vi "ezAFM Practice 1.3.vi"() -> ()   [LabVIEW 2015]
uses:
  D:/LabVIEW for ezAFM/LV-PGC 2019-05a/Special Equipment/ezAFM/NMI Integration Code/ezCommander.dll
  LabVIEW for ezAFM/LV-PGC 2019-05a/Special Equipment/ezAFM/NMI Integration Code/ezCommander.dll
  LabVIEW for ezAFM/LV-PGC 2019-05a/Universal vi's/Global Variables/Globals-EasyAFM.vi
panel:
  in  "Main Menu":enum32{"Navigation", "Scanning"}(tab)
  out "Status":string
  in  "APPROACH":bool
  in  "RETRACT":bool
  out "Retracting":bool
  out "Approaching":bool
  out "Scanning":bool
  in  "UP":bool
  in  "DOWN":bool
  in  "RIGHT":bool
  in  "LEFT":bool
  in  "Motor Speed":dbl
  in  "Step Size":dbl
  in  "Angle":dbl
  in  "THETA":bool
  out "ezAFM Connected":bool
  out "ezAFM Status":dbl
  out "XY Position":dbl[](array[numeric])
  in  "RESET":bool
  in  "MOVE":bool
  in  "Current Device":string(combo)
  in  "Target Device":string(combo)
  out "XYZ Motor Position":dbl[](array[numeric])
  out "Tip Approached?":bool
  in  "UPDATE DEVICE":bool
  out "Scan Spot":string
  out "Current Device to Scan":string
  in  "Leads":string(combo)
  in  "Device":string(combo)
  in  "Chip":string
  in  "BEGIN SCAN":bool
  in  "Image Resolution":u16(ring)=64 items=["32"=32, "64"=64, "128"=128, "256"=256, "1024"=1024, "2048"=2048]
  out "XY Vector":dbl[](array[numeric])
  in  "QUIT":bool
  # "Use Arrow Keys to manually\nmove the XY Motor"
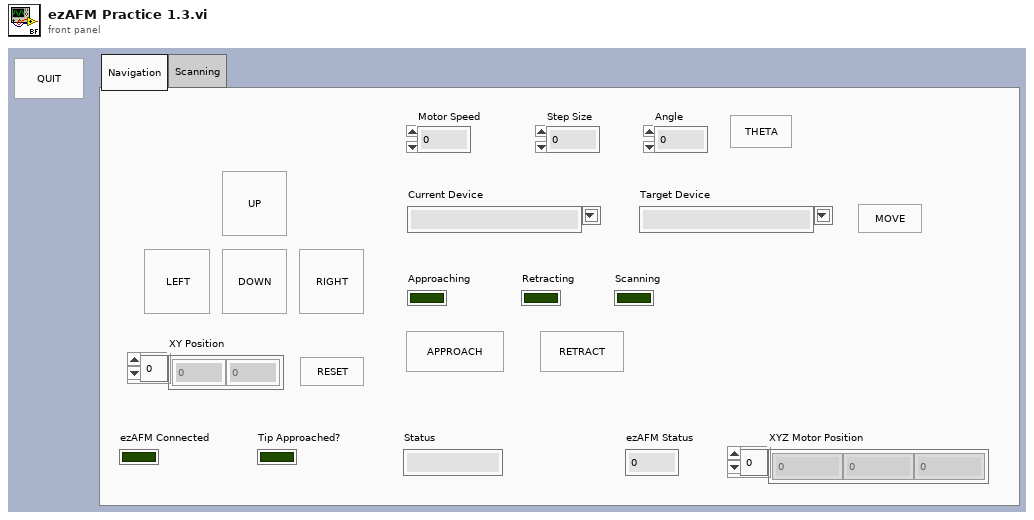
[diagram p1: front panel]
types:
  T1 = typedef "eventvkey.ctl" = enum16{"ASCII", "Enter", "Return", "Shift", "Ctrl", "Alt", "Cmd", "Opt", "Caps", "NumLock", "Clear", "Break", "Up", "Down", "Left", "Right", "Insert", "Delete", "Home", "End", "PageUp", "PageDown", "Escape", "Help", "Pause", "ScrollLock", "F1", "F2", "F3", "F4", "F5", "F6", "F7", "F8", "F9", "F10", "F11", "F12", "F13", "F14", "F15", "F16", "F17", "F18", "F19", "F20", "F21", "F22", "F23", "F24", "Play", "VolumeUp", "VolumeDown", "Mute", "Two Byte Char"}
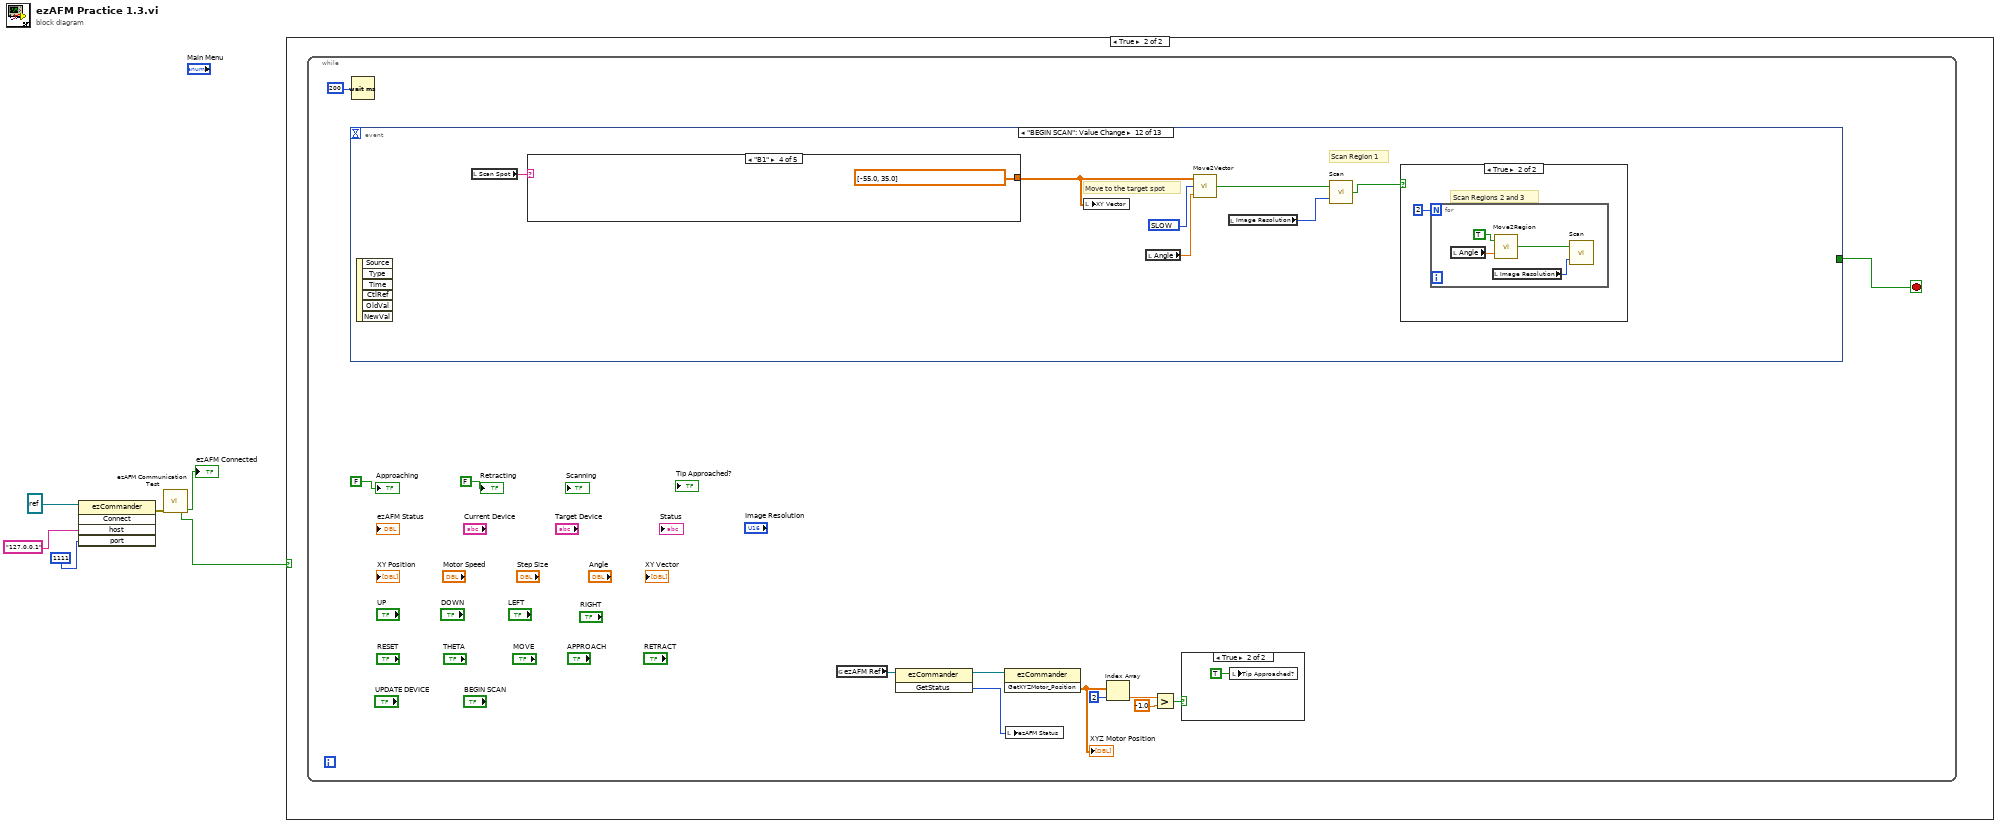
[diagram p0: block diagram]
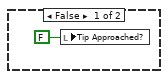
[diagram p3: hidden frame]
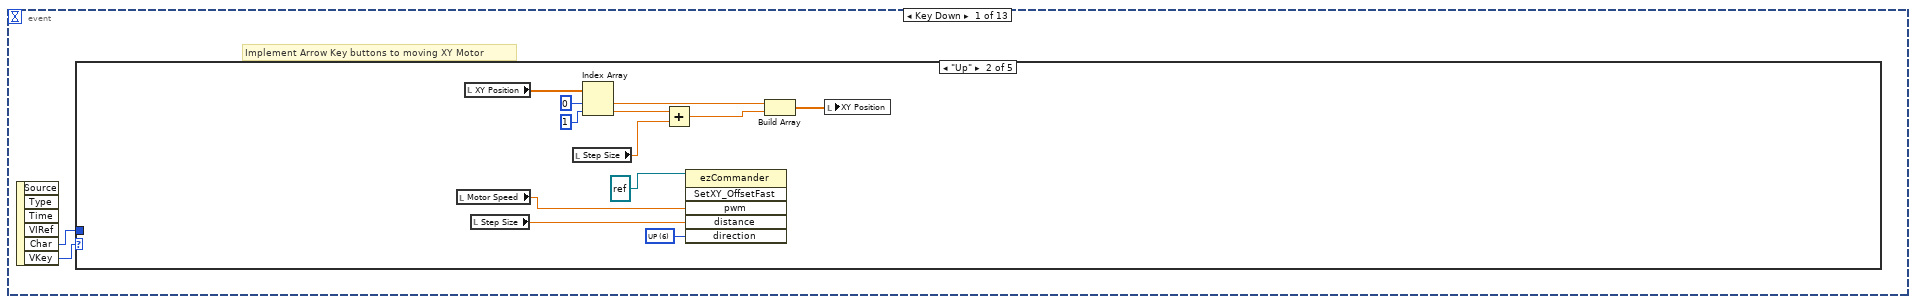
[diagram p4: hidden frame]
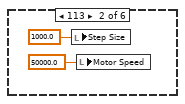
[diagram p6: hidden frame]
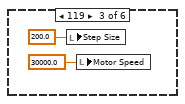
[diagram p7: hidden frame]
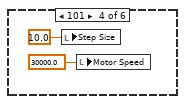
[diagram p8: hidden frame]
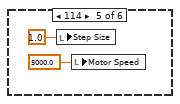
[diagram p9: hidden frame]
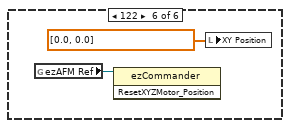
[diagram p10: hidden frame]
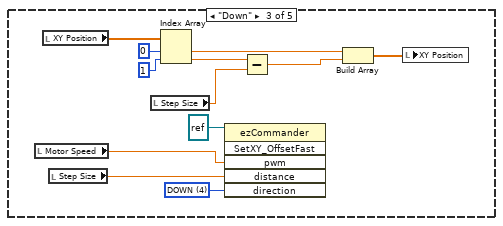
[diagram p11: hidden frame]
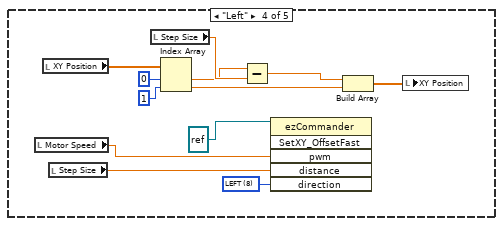
[diagram p12: hidden frame]
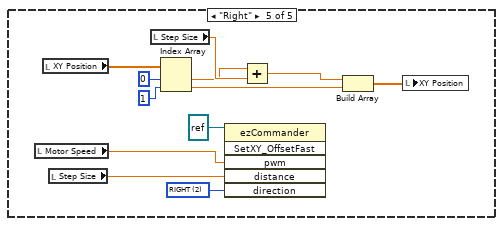
[diagram p13: hidden frame]
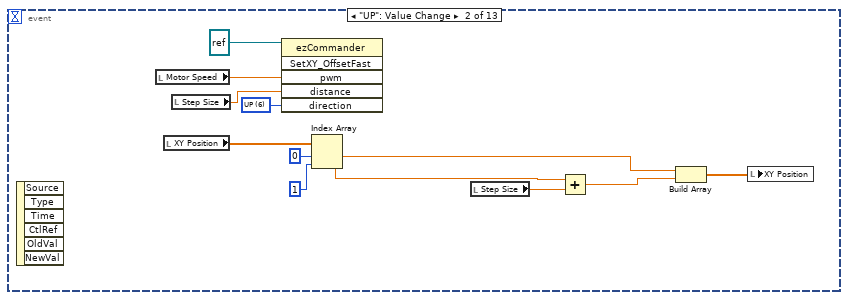
[diagram p14: hidden frame]
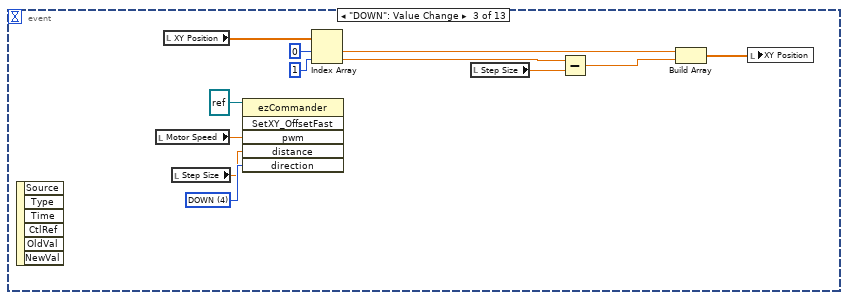
[diagram p15: hidden frame]
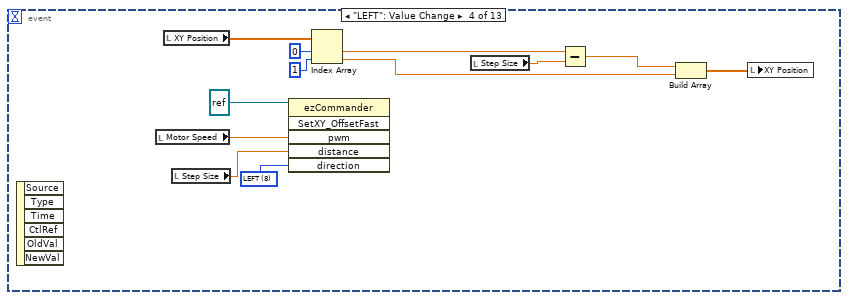
[diagram p16: hidden frame]
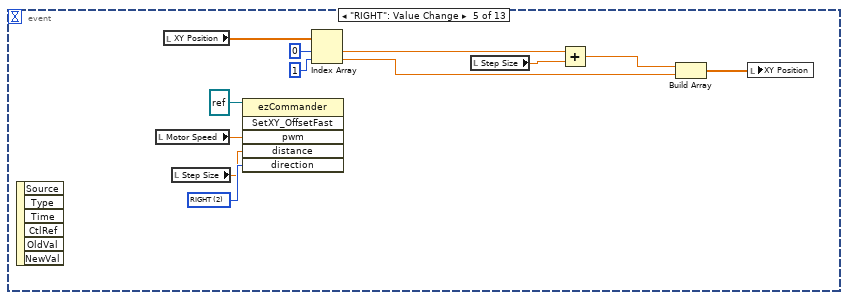
[diagram p17: hidden frame]
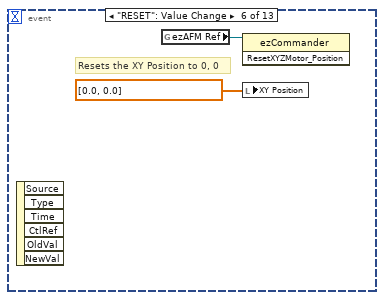
[diagram p18: hidden frame]
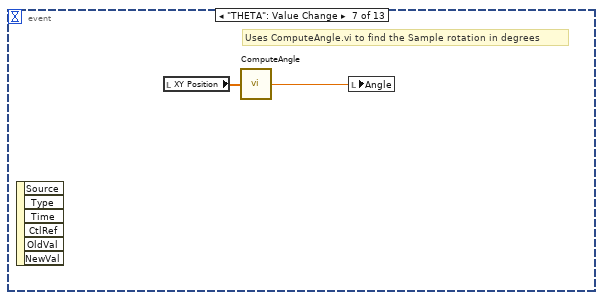
[diagram p19: hidden frame]
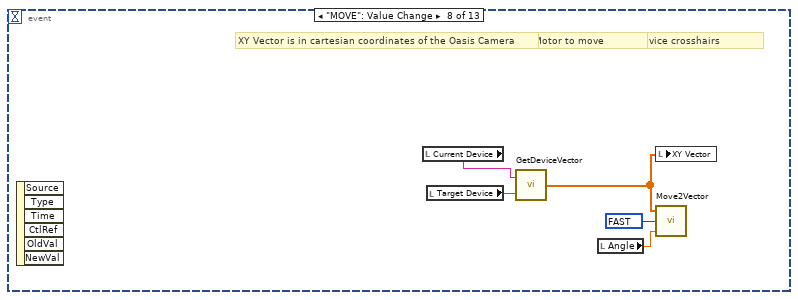
[diagram p20: hidden frame]
diagram:
  n1 = invoke class="ezCommander" method="Connect"(reference=refnum<k24> refnum ("ezAFM Ref"), "host"="127.0.0.1", "port"=1111) -> (error out=w4:errorcluster)  [unwired: 2 in, 4 out]
  n2 = call "ezAFM Communication Test.vi"("error in"=w4) -> ("ezAFM COM status"=w1:bool)  [unwired: 3 in, 3 out]
  "ezAFM Connected" <- w1
  n3 = case shown="True" w1 {
    frame False {
    }
    frame True {
      n4 = while {
        stop <- w17 stop-if-true
        n5 = event shown="[11] \"BEGIN SCAN\": Value Change" {
          selector: _ -> [_ _ _ _ _ _ _ _ _ _ _ _ _]
          dyn-events: _ -> [_ _ _ _ _ _ _ _ _ _ _ _ _]
          timeout: _ -> [_ _ _ _ _ _ _ _ _ _ _ _ _]
          tunnel: [_ _ _ _ _ _ _ _ _ _ _ _ "QUIT"] -> w17
          event Key Down {
            # "Implement Arrow Key buttons to moving XY Motor"
            n6 = event-data() -> ("Char"=w20:i16, "VKey"=w21:T1)  [unwired: 1 in, 4 out]
            n7 = case shown="\"Up\"" w21 {
              tunnel: w20 -> [w22 _ _ _ _]
              frame "ASCII", Default {
                # "Uses 'z' to reset XY Position and XYZ Motor Position"
                # "Uses 'q', 'w', 'e', 'r' keys to set different modes of movement\nAdjusts Motor Speed and Step Size"
                n8 = case shown="0, Default" w22 {
                  frame 0, Default {
                  }
                  frame 113 {
                    n9 = local write "Step Size"(1000.0 ("Step Size")) -> ()
                    n10 = local write "Motor Speed"(50000.0 ("Motor Speed")) -> ()
                  }
                  frame 119 {
                    n11 = local write "Step Size"(200.0 ("Step Size")) -> ()
                    n12 = local write "Motor Speed"(30000.0 ("Motor Speed")) -> ()
                  }
                  frame 101 {
                    n13 = local write "Step Size"(10.0 ("Step Size")) -> ()
                    n14 = local write "Motor Speed"(30000.0 ("Motor Speed")) -> ()
                  }
                  frame 114 {
                    n15 = local write "Step Size"(1.0 ("Step Size")) -> ()
                    n16 = local write "Motor Speed"(5000.0 ("Motor Speed")) -> ()
                  }
                  frame 122 {
                    n17 = global read "Globals-EasyAFM.vi" "ezAFM Ref"() -> (w31:refnum<k24>)
                    n18 = invoke class="ezCommander" method="ResetXYZMotor_Position"(reference=w31) -> ()  [unwired: 2 in, 3 out]
                    n19 = local write "XY Position"(dbl[] [0.0, 0.0] ("XY Position")) -> ()
                  }
                }
              }
              frame "Up" {
                w43 = u16 6 items=["UP"=6, "DOWN"=4, "LEFT"=8, "RIGHT"=2]
                n20 = local read "Motor Speed"() -> (w42:dbl)
                n21 = local read "XY Position"() -> (w40:dbl[])
                n22 = local read "Step Size"() -> (w41:dbl)
                n23 = local read "Step Size"() -> (w37:dbl)
                n24 = Index Array(array=w40, index #1=0 ("index"), index #2=1 ("index")) -> (element #1=w35:dbl, element #2=w36:dbl)
                n25 = Add(x=w36, y=w37) -> (x+y=w34:dbl)
                n26 = invoke class="ezCommander" method="SetXY_OffsetFast"(reference=refnum<k24> refnum ("ezAFM Ref"), "pwm"=w42, "distance"=w41, "direction"=w43) -> ()  [unwired: 2 in, 6 out]
                n27 = Build Array(w35, w34) -> (w33:dbl[])
                n28 = local write "XY Position"(w33) -> ()
              }
              frame "Down" {
                w53 = u16 4 items=["UP"=6, "DOWN"=4, "LEFT"=8, "RIGHT"=2]
                n29 = local read "Motor Speed"() -> (w55:dbl)
                n30 = local read "XY Position"() -> (w47:dbl[])
                n31 = local read "Step Size"() -> (w54:dbl)
                n32 = local read "Step Size"() -> (w46:dbl)
                n33 = Index Array(array=w47, index #1=0 ("index"), index #2=1 ("index")) -> (element #1=w49:dbl, element #2=w50:dbl)
                n34 = invoke class="ezCommander" method="SetXY_OffsetFast"(reference=refnum<k24> refnum ("ezAFM Ref"), "pwm"=w55, "distance"=w54, "direction"=w53) -> ()  [unwired: 2 in, 6 out]
                n35 = Subtract(x=w50, y=w46) -> (x-y=w48:dbl)
                n36 = Build Array(w49, w48) -> (w45:dbl[])
                n37 = local write "XY Position"(w45) -> ()
              }
              frame "Left" {
                w67 = u16 8 items=["UP"=6, "DOWN"=4, "LEFT"=8, "RIGHT"=2]
                n38 = local read "Motor Speed"() -> (w65:dbl)
                n39 = local read "XY Position"() -> (w61:dbl[])
                n40 = local read "Step Size"() -> (w66:dbl)
                n41 = local read "Step Size"() -> (w62:dbl)
                n42 = Index Array(array=w61, index #1=0 ("index"), index #2=1 ("index")) -> (element #1=w59:dbl, element #2=w57:dbl)
                n43 = Subtract(x=w59, y=w62) -> (x-y=w58:dbl)
                n44 = invoke class="ezCommander" method="SetXY_OffsetFast"(reference=refnum<k24> refnum ("ezAFM Ref"), "pwm"=w65, "distance"=w66, "direction"=w67) -> ()  [unwired: 2 in, 6 out]
                n45 = Build Array(w58, w57) -> (w60:dbl[])
                n46 = local write "XY Position"(w60) -> ()
              }
              frame "Right" {
                w79 = u16 2 items=["UP"=6, "DOWN"=4, "LEFT"=8, "RIGHT"=2]
                n47 = local read "Motor Speed"() -> (w78:dbl)
                n48 = local read "XY Position"() -> (w73:dbl[])
                n49 = local read "Step Size"() -> (w77:dbl)
                n50 = local read "Step Size"() -> (w72:dbl)
                n51 = Index Array(array=w73, index #1=0 ("index"), index #2=1 ("index")) -> (element #1=w71:dbl, element #2=w69:dbl)
                n52 = invoke class="ezCommander" method="SetXY_OffsetFast"(reference=refnum<k24> refnum ("ezAFM Ref"), "pwm"=w78, "distance"=w77, "direction"=w79) -> ()  [unwired: 2 in, 6 out]
                n53 = Add(x=w71, y=w72) -> (x+y=w70:dbl)
                n54 = Build Array(w70, w69) -> (w74:dbl[])
                n55 = local write "XY Position"(w74) -> ()
              }
            }
          }
          event "UP": Value Change {
            w91 = u16 6 items=["UP"=6, "DOWN"=4, "LEFT"=8, "RIGHT"=2]
            n56 = event-data() -> ()  [unwired: 1 in, 6 out]
            n57 = local read "Motor Speed"() -> (w84:dbl)
            n58 = local read "XY Position"() -> (w85:dbl[])
            n59 = local read "Step Size"() -> (w83:dbl)
            n60 = invoke class="ezCommander" method="SetXY_OffsetFast"(reference=refnum<k24> refnum ("ezAFM Ref"), "pwm"=w84, "distance"=w83, "direction"=w91) -> ()  [unwired: 2 in, 6 out]
            n61 = Index Array(array=w85, index #1=0 ("index"), index #2=1 ("index")) -> (element #1=w87:dbl, element #2=w88:dbl)
            n62 = local read "Step Size"() -> (w82:dbl)
            n63 = Add(x=w88, y=w82) -> (x+y=w86:dbl)
            n64 = Build Array(w87, w86) -> (w81:dbl[])
            n65 = local write "XY Position"(w81) -> ()
          }
          event "DOWN": Value Change {
            w103 = u16 4 items=["UP"=6, "DOWN"=4, "LEFT"=8, "RIGHT"=2]
            n66 = event-data() -> ()  [unwired: 1 in, 6 out]
            n67 = local read "Motor Speed"() -> (w96:dbl)
            n68 = local read "XY Position"() -> (w95:dbl[])
            n69 = local read "Step Size"() -> (w97:dbl)
            n70 = invoke class="ezCommander" method="SetXY_OffsetFast"(reference=refnum<k24> refnum ("ezAFM Ref"), "pwm"=w96, "distance"=w97, "direction"=w103) -> ()  [unwired: 2 in, 6 out]
            n71 = Index Array(array=w95, index #1=0 ("index"), index #2=1 ("index")) -> (element #1=w99:dbl, element #2=w100:dbl)
            n72 = local read "Step Size"() -> (w94:dbl)
            n73 = Subtract(x=w100, y=w94) -> (x-y=w98:dbl)
            n74 = Build Array(w99, w98) -> (w93:dbl[])
            n75 = local write "XY Position"(w93) -> ()
          }
          event "LEFT": Value Change {
            w115 = u16 8 items=["UP"=6, "DOWN"=4, "LEFT"=8, "RIGHT"=2]
            n76 = event-data() -> ()  [unwired: 1 in, 6 out]
            n77 = local read "Motor Speed"() -> (w105:dbl)
            n78 = local read "XY Position"() -> (w108:dbl[])
            n79 = local read "Step Size"() -> (w107:dbl)
            n80 = invoke class="ezCommander" method="SetXY_OffsetFast"(reference=refnum<k24> refnum ("ezAFM Ref"), "pwm"=w105, "distance"=w107, "direction"=w115) -> ()  [unwired: 2 in, 6 out]
            n81 = Index Array(array=w108, index #1=0 ("index"), index #2=1 ("index")) -> (element #1=w112:dbl, element #2=w110:dbl)
            n82 = local read "Step Size"() -> (w106:dbl)
            n83 = Subtract(x=w112, y=w106) -> (x-y=w111:dbl)
            n84 = Build Array(w111, w110) -> (w109:dbl[])
            n85 = local write "XY Position"(w109) -> ()
          }
          event "RIGHT": Value Change {
            w127 = u16 2 items=["UP"=6, "DOWN"=4, "LEFT"=8, "RIGHT"=2]
            n86 = event-data() -> ()  [unwired: 1 in, 6 out]
            n87 = local read "Motor Speed"() -> (w120:dbl)
            n88 = local read "XY Position"() -> (w119:dbl[])
            n89 = local read "Step Size"() -> (w121:dbl)
            n90 = invoke class="ezCommander" method="SetXY_OffsetFast"(reference=refnum<k24> refnum ("ezAFM Ref"), "pwm"=w120, "distance"=w121, "direction"=w127) -> ()  [unwired: 2 in, 6 out]
            n91 = Index Array(array=w119, index #1=0 ("index"), index #2=1 ("index")) -> (element #1=w124:dbl, element #2=w122:dbl)
            n92 = local read "Step Size"() -> (w118:dbl)
            n93 = Add(x=w124, y=w118) -> (x+y=w123:dbl)
            n94 = Build Array(w123, w122) -> (w117:dbl[])
            n95 = local write "XY Position"(w117) -> ()
          }
          event "RESET": Value Change {
            # "Resets the XY Position to 0, 0"
            n96 = event-data() -> ()  [unwired: 1 in, 6 out]
            n97 = global read "Globals-EasyAFM.vi" "ezAFM Ref"() -> (w129:refnum<k24>)
            n98 = invoke class="ezCommander" method="ResetXYZMotor_Position"(reference=w129) -> ()  [unwired: 2 in, 3 out]
            n99 = local write "XY Position"(dbl[] [0.0, 0.0] ("XY Position")) -> ()
          }
          event "THETA": Value Change {
            # "Uses ComputeAngle.vi to find the Sample rotation in degrees"
            n100 = event-data() -> ()  [unwired: 1 in, 6 out]
            n101 = local read "XY Position"() -> (w132:dbl[])
            n102 = call "ComputeAngle.vi"("XY Vector"=w132) -> ("Angle"=w131:dbl)
            n103 = local write "Angle"(w131) -> ()
          }
          event "MOVE": Value Change {
            w133 = u16 50000 items=["SLOW"=5000, "MEDIUM"=30000, "FAST"=50000]
            # "XY Vector is in cartesian coordinates of the Oasis Camera"
            # "Inputs the XY Vector into Move2Vector.vi to command the XY Motor to move"
            # "Uses Move2Device.vi to find the XY Vector between the Current Device and Target Device crosshairs"
            n104 = event-data() -> ()  [unwired: 1 in, 6 out]
            n105 = local read "Current Device"() -> (w136:string)
            n106 = local read "Target Device"() -> (w135:string)
            n107 = call "GetDeviceVector.vi"("Target Device"=w135, "Current Device"=w136) -> ("XY Vector"=w134:dbl[])
            n108 = local read "Angle"() -> (w137:dbl)
            n109 = local write "XY Vector"(w134) -> ()
            n110 = call "Move2Vector.vi"("Angle"=w137, "Motor Speed"=w133, "XY Vector"=w134) -> ()  [unwired: 1 out]
          }
          event "APPROACH": Value Change {
            w138 = TRUE
            n111 = event-data() -> ()  [unwired: 1 in, 6 out]
            n112 = local write "Approaching"(w138) -> ()
            n113 = call "AutoLand&Approach.vi"("Approaching?"=w138) -> ("Finished?"=w139:bool)
            n114 = local write "Tip Approached?"(w139) -> ()
          }
          event "RETRACT": Value Change {
            w140 = TRUE ("Retracting?")
            n115 = event-data() -> ()  [unwired: 1 in, 6 out]
            n116 = local write "Retracting"(w140) -> ()
            n117 = call "Retract.vi"("Number of Cycles"=10, "Retracting?"=w140) -> ("Finished?"=w142:bool)
            n118 = Not(x=w142) -> (.not. x?=w141:bool)
            n119 = local write "Tip Approached?"(w141) -> ()
          }
          event "UPDATE DEVICE": Value Change {
            n120 = event-data() -> ()  [unwired: 1 in, 6 out]
            n121 = local read "Device"() -> (w145:string)
            n122 = local read "Leads"() -> (w144:string)
            n123 = Concatenate Strings("Chip", w145, w144) -> (→"Current Device to Scan":string)
            n124 = case shown="\"abcde\"" "Leads" {
              tunnel: ["None" "A" ("string") "B" ("string")] -> w146
              frame "None", Default {
              }
              frame "abcde" {
              }
              frame "efgh" {
              }
            }
            n125 = String Length(string="Device") -> (length=w149:i32)
            n126 = Decrement(x=w149) -> (x-1=w148:i32)
            n127 = String Subset(string="Device", offset (0)=w148) -> (substring=w147:string)  [unwired: 1 in]
            n128 = case shown="\"1\", \"3\"" w147 {
              tunnel: w146 -> [w155 w157 w160]
              tunnel: [w155 w156 w159] -> w152
              frame "None", Default {
              }
              frame "0", "2" {
                n129 = Concatenate Strings(w157, "1" ("string")) -> (w156:string)
              }
              frame "1", "3" {
                n130 = Concatenate Strings(w160, "2" ("string")) -> (w159:string)
              }
            }
            "Scan Spot" <- w152
          }
          event "BEGIN SCAN": Value Change {
            w169 = u16 5000 items=["SLOW"=5000, "MEDIUM"=30000, "FAST"=50000]
            # "Scan Region 1"
            # "Move to the target spot"
            n131 = event-data() -> ()  [unwired: 1 in, 6 out]
            n132 = local read "Scan Spot"() -> (w170:string)
            n133 = case shown="\"B1\"" w170 {
              tunnel: [dbl[] [0.0, 0.0] dbl[] [-73.0, 35.0] dbl[] [-73.0, -59.0] dbl[] [-55.0, 35.0] dbl[] [-55.0, -59.0]] -> w166
              frame "None", Default {
              }
              frame "A1" {
              }
              frame "A2" {
              }
              frame "B1" {
              }
              frame "B2" {
              }
            }
            n134 = local write "XY Vector"(w166) -> ()
            n135 = local read "Angle"() -> (w168:dbl)
            n136 = call "Move2Vector.vi"("Angle"=w168, "Motor Speed"=w169, "XY Vector"=w166) -> ("Finished?"=w171:bool)
            n137 = local read "Image Resolution"() -> (w165:u16)
            n138 = call "Scan.vi"("Image Resolution"=w165, "Scanning"=w171) -> ("Finished?"=w167:bool)
            n139 = case shown="True" w167 {
              frame False {
              }
              frame True {
                # "Scan Regions 2 and 3"
                n140 = for {
                  N: 2 -> [_]
                  n141 = local read "Angle"() -> (w176:dbl)
                  n142 = local read "Image Resolution"() -> (w173:u16)
                  n143 = call "Move2Region.vi"("Angle"=w176, "Moving"=TRUE) -> ("Finished?"=w174:bool)
                  n144 = call "Scan.vi"("Image Resolution"=w173, "Scanning"=w174) -> ()  [unwired: 1 out]
                }
              }
            }
          }
          event "QUIT": Value Change {
            n145 = event-data() -> ()  [unwired: 1 in, 6 out]
          }
        }
        n146 = Wait (ms)(milliseconds to wait=u32 200) -> ()  [unwired: 1 out]
        n147 = global read "Globals-EasyAFM.vi" "ezAFM Ref"() -> (w7:refnum<k24>)
        n148 = invoke class="ezCommander" method="GetStatus"(reference=w7) -> (reference out=w6:refnum<k24>, "GetStatus"=w15:i32)  [unwired: 2 in, 1 out]
        n149 = invoke class="ezCommander" method="GetXYZMotor_Position"(reference=w6) -> ("GetXYZMotor_Position"=w8:dbl[])  [unwired: 2 in, 2 out]
        "XYZ Motor Position" <- w8
        n150 = local write "ezAFM Status"(w15) -> ()
        n151 = Index Array(array=w8, index=2) -> (element=w10:dbl)
        n152 = Greater?(x=w10, y=-1.0) -> (0:w11:bool)
        n153 = case shown="True" w11 {
          frame False {
            n154 = local write "Tip Approached?"(FALSE ("Tip Approached?")) -> ()
          }
          frame True {
            n155 = local write "Tip Approached?"(TRUE ("Tip Approached?")) -> ()
          }
        }
        "Approaching" <- FALSE ("Approaching 2")
        "Retracting" <- FALSE ("Retracting")
      }
    }
  }
